vi "calculateDelta.vi"(8 "error in (no error)":errorcluster, 11 "PeriodicWave in":refnum<class "PeriodicWave.lvclass">) -> (0 "error out":errorcluster, 2 "Delta Timestamp":dbl format="%.9f", 3 "PeriodicWave out":refnum<class "PeriodicWave.lvclass">)   [LabVIEW 2015, in "PeriodicWave.lvclass"]
uses:
  PeriodicWave.lvclass
  PeriodicWave.lvclass/PeriodicWave.ctl
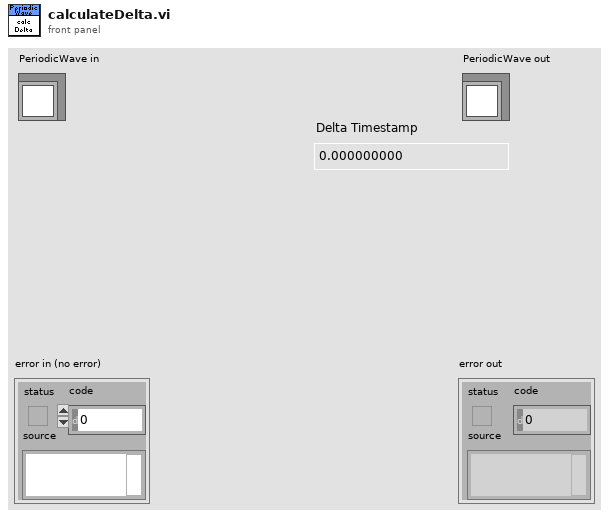
[diagram p1: front panel]
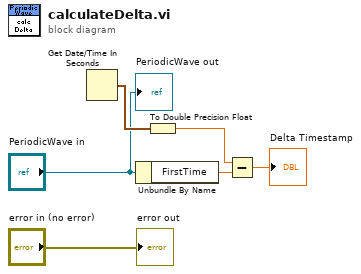
[diagram p0: block diagram]
diagram:
  n1 = Get Date/Time In Seconds() -> (seconds since 1Jan1904=w3:timestamp)
  n2 = Unbundle By Name("PeriodicWave in") -> ("FirstTime"=w4:dbl)
  n3 = To Double Precision Float(number=w3) -> (double precision float=w5:dbl)
  n4 = Subtract(x=w5, y=w4) -> (x-y=→"Delta Timestamp":dbl)
  "error out" <- "error in (no error)"
  "PeriodicWave out" <- "PeriodicWave in"
